vi "SinCos.vi"(1 "SinCos":refnum<class "SinCos.lvclass">, 7 "X":sgl) -> (6 "sinX":sgl, 10 "cosX":sgl)   [LabVIEW 2017, in "SinCos.lvclass"]
uses:
  SinCos.lvclass
  <vilib>/rvi/FXPMathLib/FxpSinAndCos/subVIs/nifxpmath_SinAndCos_SimConfig.ctl
  <vilib>/rvi/FXPMathLib/FxpSinAndCos/simVIs/DllFxpSinAndCosTemp_sub.vi
  <vilib>/rvi/FXPMathLib/FxpSinAndCos/XNode/nifxpmath_SinAndCos.xnode
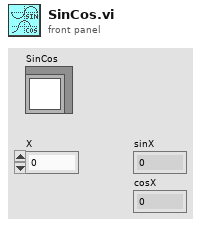
[diagram p1: front panel]
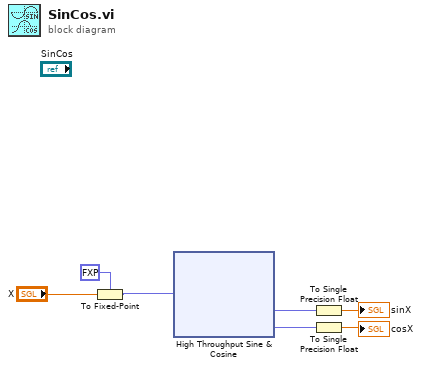
[diagram p0: block diagram]
diagram:
  n1 = To Fixed-Point(fixed-point type=fxp<+/-,16,1> 0.0 ("x (pi)"), number="X") -> (fixed-point=w1:fxp<+/-,16,1>)
  n2 = xnode "High Throughput Sine & Cosine"("x (pi)"=w1) -> ("sin(x)"=w7:fxp<+/-,16,2>, "cos(x)"=w6:fxp<+/-,16,2>)
  n3 = To Single Precision Float(number=w7) -> (single precision float=→"sinX":sgl)
  n4 = To Single Precision Float(number=w6) -> (single precision float=→"cosX":sgl)
